vi "Read View Settings Event Ref.vi"(8 "error in (no error)":errorcluster, 11 "Controller Actor in":refnum<class "Controller Actor.lvclass">) -> (0 "error out":errorcluster, 2 "View Settings Event Ref":T1, 3 "Controller Actor out":refnum<class "Controller Actor.lvclass">)   [LabVIEW 2016, in "Event Actors.lvlib" / "Controller Actor.lvclass"]
uses:
  Controller Actor.lvclass
  View Settings Event Ref.ctl
  View Settings.ctl
  Controller Actor.lvclass/Controller Actor.ctl
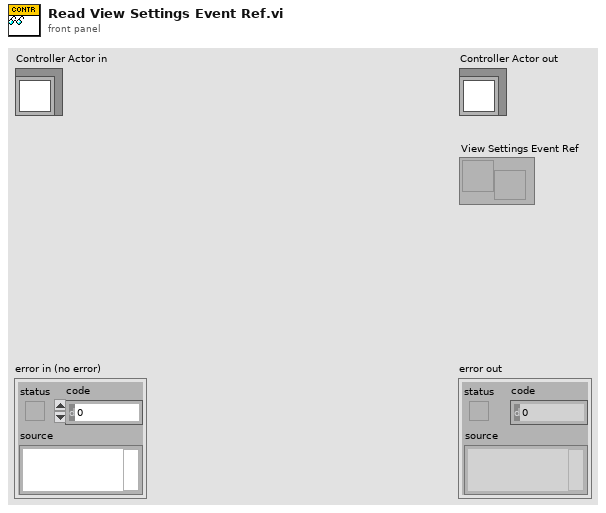
[diagram p1: front panel]
types:
  T1 = typedef "Event Actors.lvlib/Controller Actor.lvclass/View Settings Event Ref.ctl" = refnum<user-event>
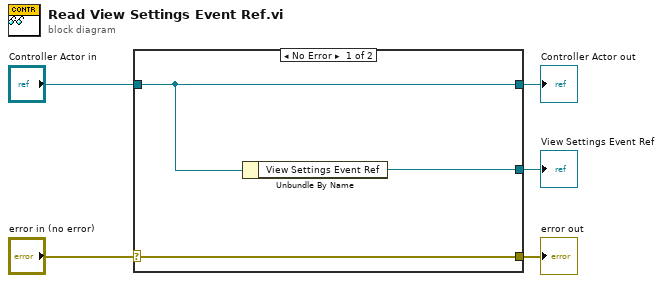
[diagram p0: block diagram]
diagram:
  n1 = case shown="No Error" "error in (no error)" {
    selector: "error in (no error)" -> [w8 w9]
    tunnel: [w8 w9] -> w4
    tunnel: [w7 w10] -> w2
    tunnel: "Controller Actor in" -> [w7 w10]
    tunnel: [w6 _] -> w1
    frame No Error {
      n2 = Unbundle By Name(w7) -> ("View Settings Event Ref"=w6:T1)
    }
    frame Error {
    }
  }
  "error out" <- w4
  "Controller Actor out" <- w2
  "View Settings Event Ref" <- w1
